vi "tx streamer recv async msg.vi"(7 "valid":i32, 8 "error in (no error)":errorcluster, 9 "timeout":dbl, 10 "md":u64, 11 "h":u64) -> (0 "error out":errorcluster, 2 "md out":u64, 3 "function return":u32(ring), 5 "valid out":i32)   [LabVIEW 2023, in "uhd.lvlib"]
doc: "UHD_API uhd_error uhd_tx_streamer_recv_async_msg(\n uhd_tx_streamer_handle h, uhd_async_metadata_handle* md, double timeout, bool* valid);"
uses:
  <userlib>/uhd/uhd.lvlib
  <userlib>/uhd/uhd.dll
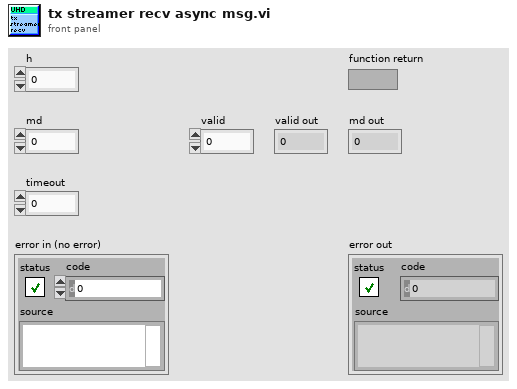
[diagram p1: front panel]
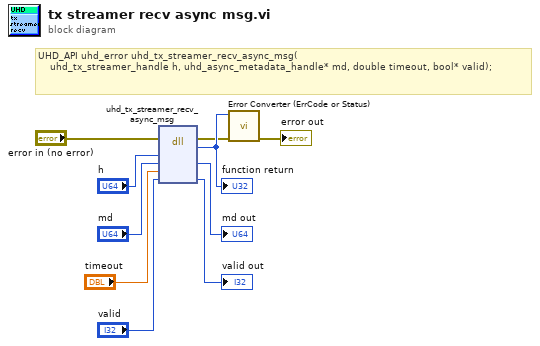
[diagram p0: block diagram]
diagram:
  # "UHD_API uhd_error uhd_tx_streamer_recv_async_msg(\n    uhd_tx_streamer_handle h, uhd_async_metadata_handle* md, double timeout, bool* valid);"
  n1 = dll-call lib="C:/Program Files/National Instruments/LabVIEW 2023/user.lib/uhd/uhd.*" fn="uhd_tx_streamer_recv_async_msg"(error in="error in (no error)", "h"="h", "md"="md", "timeout"="timeout", "valid"="valid") -> (error out=w2:errorcluster, w10:u32, "md"=→"md out":u64, "valid"=→"valid out":i32)  [unwired: 4 in, 1 out]
  "function return" <- w10
  n2 = call <userlib>:"Error Converter (ErrCode or Status).vi"("error in (no error)"=w2, "error code"=w10) -> ("error out"=→"error out":errorcluster)  [unwired: 9 in]
